vi "Write Status Msg.vi"(8 "error in (no error)":errorcluster, 10 "Proxy.lvlib:Proxy Status Msg.lvclass":refnum<class "Proxy Status Msg.lvclass">, 11 "Proxy in":refnum<class "Proxy.lvclass">) -> (0 "error out":errorcluster, 3 "Proxy out":refnum<class "Proxy.lvclass">)   [LabVIEW 2014, in "Proxy.lvlib" / "Proxy.lvclass"]
uses:
  Proxy.lvclass
  Proxy Messages/Proxy Status Msg/Proxy Status Msg.lvclass
  Proxy.lvclass/Proxy.ctl
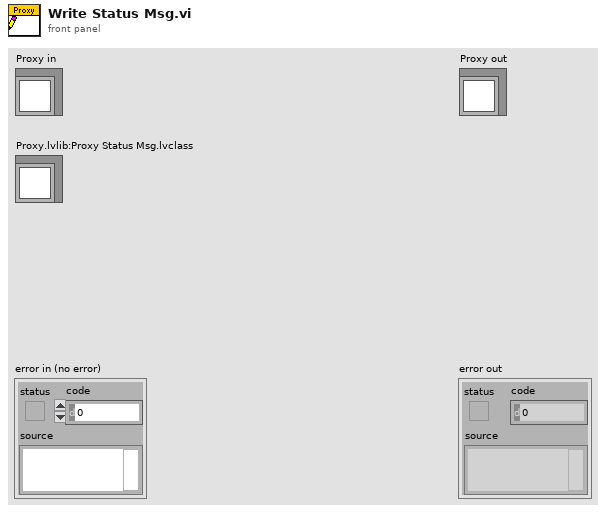
[diagram p1: front panel]
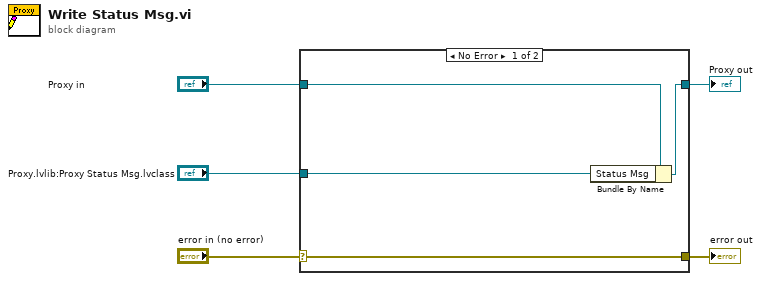
[diagram p0: block diagram]
diagram:
  n1 = case shown="No Error" "error in (no error)" {
    selector: "error in (no error)" -> [w9 w10]
    tunnel: [w9 w10] -> w4
    tunnel: [w7 w11] -> w2
    tunnel: "Proxy in" -> [w8 w11]
    tunnel: "Proxy.lvlib:Proxy Status Msg.lvclass" -> [w6 _]
    frame No Error {
      n2 = Bundle By Name(cluster=w8, "Status Msg"=w6) -> (w7:refnum<class "Proxy.lvclass">)
    }
    frame Error {
    }
  }
  "error out" <- w4
  "Proxy out" <- w2
